vi "Destroy.vi"(8 "error in (no error)":errorcluster, 11 "MJPEG Reader in":refnum<data-value>) -> (0 "error out":errorcluster)   [LabVIEW 2015, in "MJPEG Reader.lvclass"]
doc: "Destroys the MJPEG Reader and closes internal references."
uses:
  MJPEG Reader.lvclass
  MJPEG Reader.lvclass/MJPEG Reader.ctl
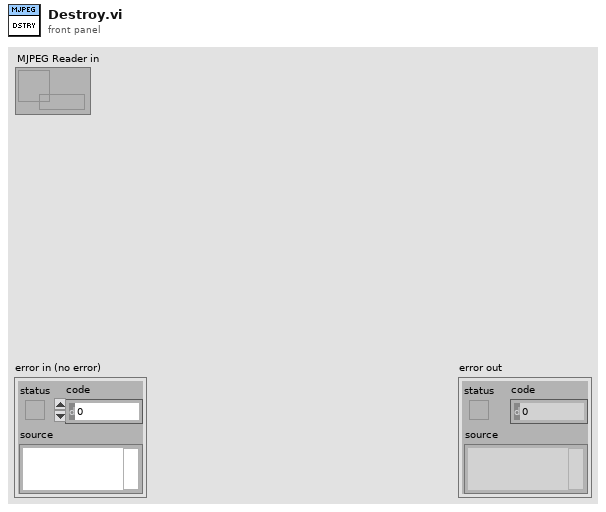
[diagram p1: front panel]
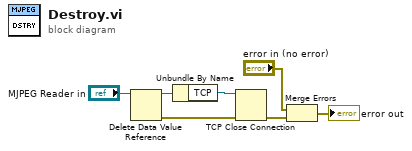
[diagram p0: block diagram]
diagram:
  n1 = Delete Data Value Reference(data value reference="MJPEG Reader in") -> (data value=w6:refnum<class "MJPEG Reader.lvclass">, error out=w4:errorcluster)  [unwired: 1 in]
  n2 = Unbundle By Name(w6) -> ("TCP"=w5:refnum<k5>)
  n3 = TCP Close Connection(connection ID=w5, error in (no error)=w4) -> (error out=w2:errorcluster)  [unwired: 1 in, 1 out]
  n4 = Merge Errors("error in (no error)", w2) -> (→"error out":errorcluster)
